vi "Enumerate Ports.vi"(8 "list?":bool=TRUE, 9 "Processor":T1, 11 "Python version":string="3.9") -> (0 "error out":errorcluster, 1 "guess":string, 3 "Python":T2, 4 "name":string, 5 "possibilities":string[](array[string]))   [LabVIEW 2021]
uses:
  PythonCtrl.ctl
  LabVIEWOpenMV/_subs/Processors.ctl
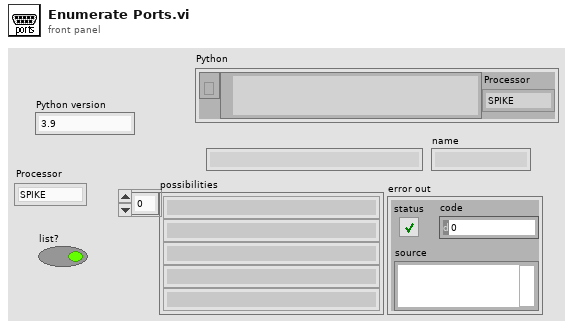
[diagram p1: front panel]
types:
  T1 = typedef "Processors.ctl" = enum16{"SPIKE", "Pi", "Pi_ssh", "OpenMV"}
  T2 = typedef "PythonCtrl.ctl" = cluster{"session":refnum<k35>, "PyPath":path, "Processor":T1}
  T3 = cluster{"Refnum out":refnum<k35>, "appended path":path, "Processor":T1}
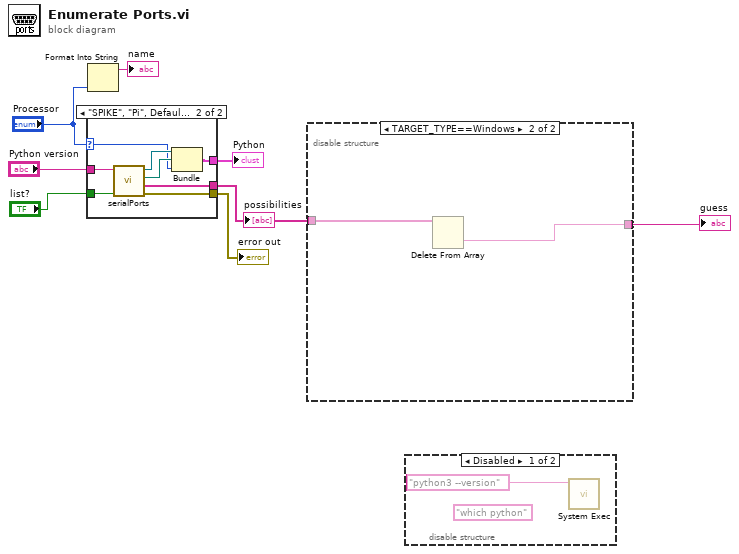
[diagram p0: block diagram]
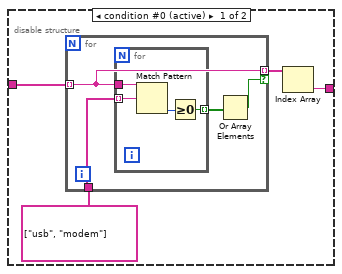
[diagram p2: hidden frame]
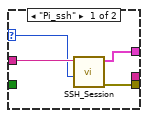
[diagram p3: hidden frame]
diagram:
  n1 = case shown="\"SPIKE\", \"Pi\", Default" "Processor" {
    selector: "Processor" -> [w9 w14]
    tunnel: [_ w20] -> w7
    tunnel: [w10 w19] -> w5
    tunnel: "Python version" -> [w12 w18]
    tunnel: [w11 w15] -> w2
    tunnel: "list?" -> [_ w13]
    frame "Pi_ssh" {
      n2 = call "SSH_Session.vi"("Processor"=w9, "Python version"=w12) -> ("error out"=w10:errorcluster, "Python"=w11:T2)  [unwired: 8 in]
    }
    frame "SPIKE", "Pi", Default {
      n3 = call "serialPorts.vi"("list?"=w13, "Python version"=w18) -> ("error out"=w19:errorcluster, "ports"=w20:string[], "appended path"=w16:path, "Refnum out"=w17:refnum<k35>)  [unwired: 6 in]
      n4 = Bundle("Refnum out"=w17, "appended path"=w16, "Processor"=w14) -> (w15:T3)  [unwired: 1 in]
    }
  }
  "possibilities" <- w7
  "error out" <- w5
  "Python" <- w2
  n5 = Format Into String("Processor") -> (resulting string=→"name":string)  [unwired: 3 in, 1 out]
  n6 = disable-structure shown="TARGET_TYPE==Windows" {
    disable-tunnel: [w23 w33] -> w8
    disable-tunnel: w7 -> [w22 w34]
    frame condition #0 (active) {
      n7 = for {
        tunnel: w22 -> [w26] mode=indexing
        tunnel: string[] ["usb", "modem"] -> [w28]
        tunnel: [w26] -> w21 mode=indexing if=w25
        n8 = for {
          tunnel: w26 -> [w32]
          tunnel: w28 -> [w31] mode=indexing
          tunnel: [w29] -> w27 mode=indexing
          n9 = Match Pattern(string=w32, regular expression=w31) -> (offset past match=w30:i32)  [unwired: 1 in, 3 out]
          n10 = Greater Or Equal To 0?(x=w30) -> (x >= 0?=w29:bool)
        }
        n11 = Or Array Elements(Boolean array=w27) -> (logical OR=w25:bool)
      }
      n12 = Index Array(array=w21) -> (element=w23:string)  [unwired: 1 in]
    }
    frame condition #1 {
      n13 = Delete From Array(array=w34) -> (deleted portion=w33:string)  [unwired: 2 in, 1 out]
    }
  }
  "guess" <- w8
  n14 = disable-structure shown="Disabled" {
    frame Disabled {
      (unwired) "which python" ("command line")
      n15 = call <vilib>:"System Exec.vi"("command line"="python3 --version") -> ()  [unwired: 7 in, 4 out]
    }
    frame Enabled {
    }
  }
